vi "Registry Set.vi"() -> (0 "error out":errorcluster)   [LabVIEW 2012]
uses:
  <vilib>/Rock Robotics/WPI/Joystick/WPI_JoystickDeviceEnum.ctl
  <vilib>/Rock Robotics/SystemInterfaces/AI/FPGA_AIChannel.ctl
  <vilib>/Rock Robotics/SystemInterfaces/Typedef/FPGA_TypedefAnalogModule.ctl
  <vilib>/Rock Robotics/SystemInterfaces/DIO/FPGA_DIOPWMChannel.ctl
  <vilib>/Rock Robotics/SystemInterfaces/Typedef/FPGA_TypedefDigitalModule.ctl
  <vilib>/Rock Robotics/SystemInterfaces/DIO/FPGA_DIOChannel.ctl
  <vilib>/Rock Robotics/SystemInterfaces/DIO/FPGA_DIORelayChannel.ctl
  <vilib>/Rock Robotics/WPI/Solenoid/WPI_SolenoidChannel.ctl
  <vilib>/Rock Robotics/SystemInterfaces/Typedef/FPGA_TypedefSolenoidModule.ctl
  <vilib>/Rock Robotics/WPI/MotorControl/WPI_MotorControlOpen Talon.vi
  <vilib>/Rock Robotics/WPI/Solenoid/WPI_SolenoidOpenSingle.vi
  <vilib>/Rock Robotics/WPI/Solenoid/WPI_SolenoidOpenDouble.vi
  Global Refnums.vi
  <vilib>/Rock Robotics/WPI/Compressor/WPI_CompressorGetSetRefNum.vi
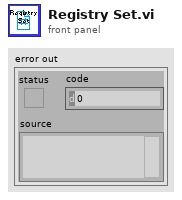
[diagram p1: front panel]
types:
  T1 = typedef "WPI_SolenoidChannel.ctl" = enum8{"Solenoid 1", "Solenoid 2", "Solenoid 3", "Solenoid 4", "Solenoid 5", "Solenoid 6", "Solenoid 7", "Solenoid 8", "Invalid"}
  T2 = typedef "FPGA_TypedefSolenoidModule.ctl" = enum16{"Solenoid Module 1", "Solenoid Module 2"}
  T3 = typedef "FPGA_DIOChannel.ctl" = enum8{"DIO 1", "DIO 2", "DIO 3", "DIO 4", "DIO 5", "DIO 6", "DIO 7", "DIO 8", "DIO 9", "DIO 10", "DIO 11", "DIO 12", "DIO 13", "DIO 14", "Invalid"}
  T4 = typedef "FPGA_TypedefDigitalModule.ctl" = enum16{"Digital Module 1", "Digital Module 2"}
  T5 = typedef "FPGA_DIOPWMChannel.ctl" = enum8{"PWM 1", "PWM 2", "PWM 3", "PWM 4", "PWM 5", "PWM 6", "PWM 7", "PWM 8", "PWM 9", "PWM 10", "Invalid"}
  T6 = typedef "FPGA_DIORelayChannel.ctl" = enum8{"Relay 1", "Relay 2", "Relay 3", "Relay 4", "Relay 5", "Relay 6", "Relay 7", "Relay 8", "Invalid"}
  T7 = typedef "FPGA_AIChannel.ctl" = enum8{"AI 1", "AI 2", "AI 3", "AI 4", "AI 5", "AI 6", "AI 7", "AI 8", "Invalid"}
  T8 = typedef "FPGA_TypedefAnalogModule.ctl" = enum16{"Analog Module 1", "Analog Module 2"}
  T9 = typedef "WPI_JoystickDeviceEnum.ctl" = enum16{"USB 1", "USB 2", "USB 3", "USB 4", "Kinect 1", "Kinect 2"}
  T10 = typedef "WPI_AnalogChannelDevRef.ctl" = cluster{"DevStatus":errorcluster, "Analog Module":T8, "Analog Channel":T7}
  T11 = typedef "WPI_JoystickDevRef.ctl" = cluster{"Device":T9}
  T12 = typedef "WPI_CompressorDevRef.ctl" = cluster{"DevStatus":errorcluster, "DigitalInputDevRef":T13, "RelayDevRef":T14}
  T13 = typedef "WPI_DigitalInputDevRef.ctl" = cluster{"DevStatus":errorcluster, "DIO Channel":T3, "Digital Module":T4}
  T14 = typedef "WPI_RelayDevRef.ctl" = cluster{"DevStatus":errorcluster, "Relay Channel":T6, "Digital Module":T4, "Relay Direction":T15}
  T15 = typedef "WPI_RelayDirection.ctl" = enum16{"Both directions", "Forward only", "Reverse only"}
  T16 = typedef "WPI_MotorControlDeviceRef.ctl" = cluster{"DeviceStatus":errorcluster, "Type":enum16{"PWM", "CAN"}, "PWM":cluster{"Digital Module":T4, "PWM Channel":T5, "DeadBand":T17}, "CAN":cluster{"Device Number":u8, "Control Mode":T18, "Semaphore":T19, "Max Vout":dbl}, "Invert":bool, "TransformRef":T20, "InvTransformRef":T20}
  T17 = typedef "WPI_PWMDeadband.ctl" = cluster{"Name":string, "maxPositivePwm":i32, "minPositivePwm":i32, "centerPwm":i32, "maxNegativePwm":i32, "minNegativePwm":i32, "angularRange":u16}
  T18 = typedef "WPI_CANJaguar_ControlMode.ctl" = enum8{"Percent VBus", "Current", "Speed", "Position", "Voltage"}
  T19 = typedef "Semaphore RefNum" = refnum<k1>
  T20 = typedef "WPI_PWMTransform_ConPane.ctl" = refnum<vi>
  T21 = typedef "WPI_SolenoidDevRef.ctl" = cluster{"DevStatus":errorcluster, "Solenoid Module":T2, "Forward Solenoid Channel":T1, "Reverse Solenoid Channel":T1}
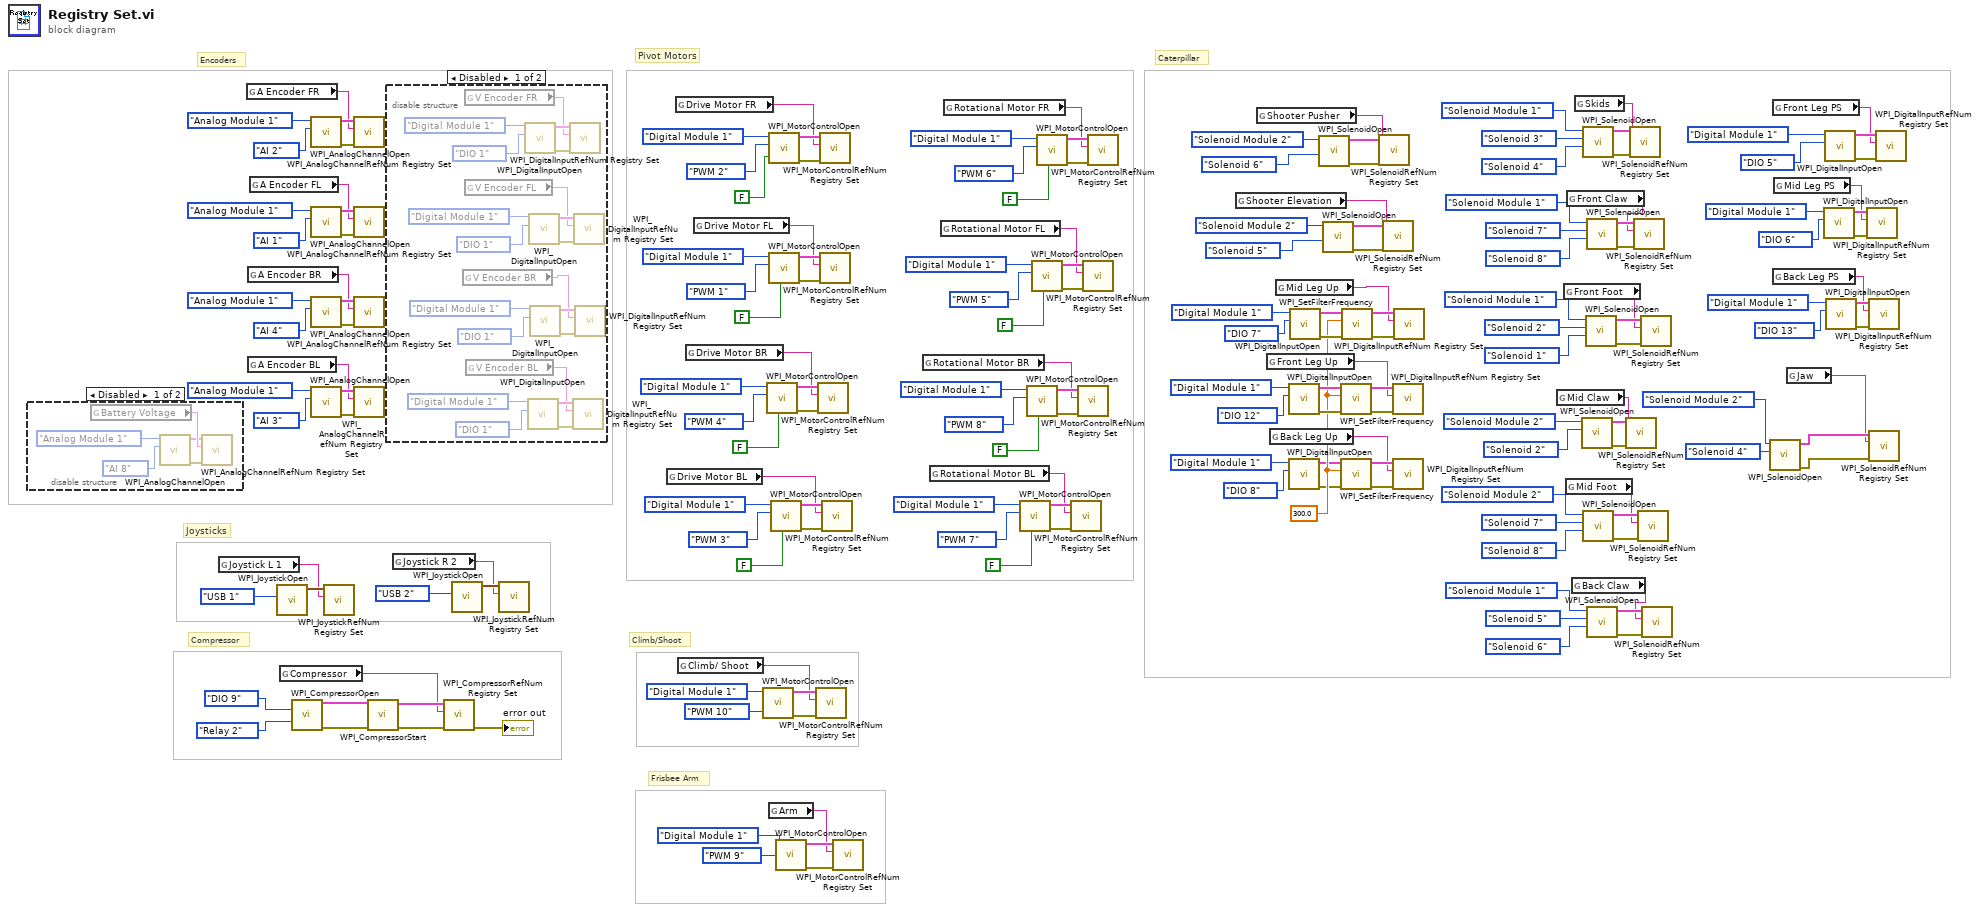
[diagram p0: block diagram]
diagram:
  w91 = 300.0 ("Filter Frequency")
  # "Frisbee Arm"
  # "Compressor"
  # "Climb/Shoot"
  # "Caterpillar"
  # "Pivot Motors"
  # "Encoders"
  # "Joysticks"
  n1 = disable-structure shown="Disabled" {
    frame Disabled {
      n2 = global read "Global Refnums.vi" "Battery Voltage"() -> (w184:string)
      n3 = call <vilib>:"WPI_AnalogChannelOpen.vi"("Analog Channel"=FPGA_AIChannel."AI 8", "Analog Module (Module 1)"=FPGA_TypedefAnalogModule."Analog Module 1") -> ("error out"=w181:errorcluster, "AIDeviceRef"=w180:T10)  [unwired: 8 in]
      n4 = call <vilib>:"WPI_AnalogChannelRefNum Registry Set.vi"("error in (no error)"=w181, "refnum name"=w184, "AIDeviceRef"=w180) -> ()  [unwired: 7 in, 2 out]
    }
    frame Enabled {
    }
  }
  n5 = global read "Global Refnums.vi" "Joystick L 1"() -> (w177:string)
  n6 = global read "Global Refnums.vi" "A Encoder FR"() -> (w169:string)
  n7 = global read "Global Refnums.vi" "A Encoder BR"() -> (w155:string)
  n8 = global read "Global Refnums.vi" "A Encoder BL"() -> (w154:string)
  n9 = global read "Global Refnums.vi" "A Encoder FL"() -> (w156:string)
  n10 = call <vilib>:"WPI_JoystickOpen.vi"("JoystickDevice"=WPI_JoystickDeviceEnum."USB 1") -> ("JoystickDevRef"=w178:T11)  [unwired: 10 in]
  n11 = global read "Global Refnums.vi" "Compressor"() -> (w80:string)
  n12 = call <vilib>:"WPI_CompressorOpen.vi"("Pressure Switch DIO Channel"=FPGA_DIOChannel."DIO 9", "Relay Channel"=FPGA_DIORelayChannel."Relay 2") -> ("CompressorDevRef"=w86:T12, "error out"=w85:errorcluster)  [unwired: 12 in]
  n13 = call <vilib>:"WPI_AnalogChannelOpen.vi"("Analog Channel"=FPGA_AIChannel."AI 2", "Analog Module (Module 1)"=FPGA_TypedefAnalogModule."Analog Module 1") -> ("error out"=w172:errorcluster, "AIDeviceRef"=w173:T10)  [unwired: 8 in]
  n14 = call <vilib>:"WPI_AnalogChannelOpen.vi"("Analog Channel"=FPGA_AIChannel."AI 1", "Analog Module (Module 1)"=FPGA_TypedefAnalogModule."Analog Module 1") -> ("error out"=w167:errorcluster, "AIDeviceRef"=w168:T10)  [unwired: 8 in]
  n15 = call <vilib>:"WPI_AnalogChannelOpen.vi"("Analog Channel"=FPGA_AIChannel."AI 4", "Analog Module (Module 1)"=FPGA_TypedefAnalogModule."Analog Module 1") -> ("error out"=w163:errorcluster, "AIDeviceRef"=w164:T10)  [unwired: 8 in]
  n16 = call <vilib>:"WPI_AnalogChannelOpen.vi"("Analog Channel"=FPGA_AIChannel."AI 3", "Analog Module (Module 1)"=FPGA_TypedefAnalogModule."Analog Module 1") -> ("error out"=w159:errorcluster, "AIDeviceRef"=w160:T10)  [unwired: 8 in]
  n17 = call <vilib>:"WPI_JoystickRefNum Registry Set.vi"("refnum name"=w177, "JoystickDevRef"=w178) -> ()  [unwired: 8 in, 2 out]
  n18 = call <vilib>:"WPI_AnalogChannelRefNum Registry Set.vi"("error in (no error)"=w172, "refnum name"=w169, "AIDeviceRef"=w173) -> ()  [unwired: 7 in, 2 out]
  n19 = call <vilib>:"WPI_AnalogChannelRefNum Registry Set.vi"("error in (no error)"=w167, "refnum name"=w156, "AIDeviceRef"=w168) -> ()  [unwired: 7 in, 2 out]
  n20 = call <vilib>:"WPI_AnalogChannelRefNum Registry Set.vi"("error in (no error)"=w163, "refnum name"=w155, "AIDeviceRef"=w164) -> ()  [unwired: 7 in, 2 out]
  n21 = call <vilib>:"WPI_AnalogChannelRefNum Registry Set.vi"("error in (no error)"=w159, "refnum name"=w154, "AIDeviceRef"=w160) -> ()  [unwired: 7 in, 2 out]
  n22 = call <vilib>:"WPI_CompressorStart.vi"("error in (no error)"=w85, "CompressorDevRef"=w86) -> ("error out"=w83:errorcluster, "CompressorDevRef"=w84:T12)  [unwired: 8 in]
  n23 = disable-structure shown="Disabled" {
    frame Disabled {
      n24 = global read "Global Refnums.vi" "V Encoder BR"() -> (w190:string)
      n25 = global read "Global Refnums.vi" "V Encoder FR"() -> (w202:string)
      n26 = global read "Global Refnums.vi" "V Encoder FL"() -> (w195:string)
      n27 = global read "Global Refnums.vi" "V Encoder BL"() -> (w185:string)
      n28 = call <vilib>:"WPI_DigitalInputOpen.vi"("DIO Channel"=FPGA_DIOChannel."DIO 1", "Digital Module (Module 1)"=FPGA_TypedefDigitalModule."Digital Module 1") -> ("error out"=w204:errorcluster, "DigitalInputDevRef"=w203:T13)  [unwired: 8 in]
      n29 = call <vilib>:"WPI_DigitalInputOpen.vi"("DIO Channel"=FPGA_DIOChannel."DIO 1", "Digital Module (Module 1)"=FPGA_TypedefDigitalModule."Digital Module 1") -> ("error out"=w189:errorcluster, "DigitalInputDevRef"=w188:T13)  [unwired: 8 in]
      n30 = call <vilib>:"WPI_DigitalInputOpen.vi"("DIO Channel"=FPGA_DIOChannel."DIO 1", "Digital Module (Module 1)"=FPGA_TypedefDigitalModule."Digital Module 1") -> ("error out"=w199:errorcluster, "DigitalInputDevRef"=w198:T13)  [unwired: 8 in]
      n31 = call <vilib>:"WPI_DigitalInputOpen.vi"("DIO Channel"=FPGA_DIOChannel."DIO 1", "Digital Module (Module 1)"=FPGA_TypedefDigitalModule."Digital Module 1") -> ("error out"=w194:errorcluster, "DigitalInputDevRef"=w193:T13)  [unwired: 8 in]
      n32 = call <vilib>:"WPI_DigitalInputRefNum Registry Set.vi"("error in (no error)"=w204, "refnum name"=w202, "DigitalInputDevRef"=w203) -> ()  [unwired: 7 in, 2 out]
      n33 = call <vilib>:"WPI_DigitalInputRefNum Registry Set.vi"("error in (no error)"=w189, "refnum name"=w185, "DigitalInputDevRef"=w188) -> ()  [unwired: 7 in, 2 out]
      n34 = call <vilib>:"WPI_DigitalInputRefNum Registry Set.vi"("error in (no error)"=w199, "refnum name"=w195, "DigitalInputDevRef"=w198) -> ()  [unwired: 7 in, 2 out]
      n35 = call <vilib>:"WPI_DigitalInputRefNum Registry Set.vi"("error in (no error)"=w194, "refnum name"=w190, "DigitalInputDevRef"=w193) -> ()  [unwired: 7 in, 2 out]
    }
    frame Enabled {
    }
  }
  n36 = global read "Global Refnums.vi" "Joystick R 2"() -> (w174:string)
  n37 = call <vilib>:"WPI_CompressorRefNum Registry Set.vi"("error in (no error)"=w83, "refnum name"=w80, "CompressorDevRef"=w84) -> ("error out"=→"error out":errorcluster)  [unwired: 7 in, 1 out]
  n38 = call <vilib>:"WPI_JoystickOpen.vi"("JoystickDevice"=WPI_JoystickDeviceEnum."USB 2") -> ("JoystickDevRef"=w175:T11)  [unwired: 10 in]
  n39 = call <vilib>:"WPI_JoystickRefNum Registry Set.vi"("refnum name"=w174, "JoystickDevRef"=w175) -> ()  [unwired: 8 in, 2 out]
  n40 = global read "Global Refnums.vi" "Drive Motor BL"() -> (w131:string)
  n41 = global read "Global Refnums.vi" "Drive Motor FR"() -> (w149:string)
  n42 = global read "Global Refnums.vi" "Climb/ Shoot"() -> (w32:string)
  n43 = global read "Global Refnums.vi" "Drive Motor BR"() -> (w130:string)
  n44 = global read "Global Refnums.vi" "Drive Motor FL"() -> (w137:string)
  n45 = call-poly <vilib>:"WPI_MotorControlOpen.vi"("PWM Channel"=FPGA_DIOPWMChannel."PWM 10", "Digital Module (Module 1)"=FPGA_TypedefDigitalModule."Digital Module 1") -> ("error out"=w35:errorcluster, "MotorControlDeviceRef"=w36:T16)  [unwired: 8 in]
  n46 = call-poly <vilib>:"WPI_MotorControlOpen.vi"("Invert"=FALSE, "PWM Channel"=FPGA_DIOPWMChannel."PWM 4", "Digital Module (Module 1)"=FPGA_TypedefDigitalModule."Digital Module 1") -> ("error out"=w139:errorcluster, "MotorControlDeviceRef"=w140:T16)  [unwired: 7 in]
  n47 = call-poly <vilib>:"WPI_MotorControlOpen.vi"("Invert"=FALSE, "PWM Channel"=FPGA_DIOPWMChannel."PWM 2", "Digital Module (Module 1)"=FPGA_TypedefDigitalModule."Digital Module 1") -> ("error out"=w150:errorcluster, "MotorControlDeviceRef"=w151:T16)  [unwired: 7 in]
  n48 = call-poly <vilib>:"WPI_MotorControlOpen.vi"("Invert"=FALSE, "PWM Channel"=FPGA_DIOPWMChannel."PWM 1", "Digital Module (Module 1)"=FPGA_TypedefDigitalModule."Digital Module 1") -> ("error out"=w144:errorcluster, "MotorControlDeviceRef"=w145:T16)  [unwired: 7 in]
  n49 = global read "Global Refnums.vi" "Arm"() -> (w18:string)
  n50 = call-poly <vilib>:"WPI_MotorControlOpen.vi"("Invert"=FALSE, "PWM Channel"=FPGA_DIOPWMChannel."PWM 3", "Digital Module (Module 1)"=FPGA_TypedefDigitalModule."Digital Module 1") -> ("error out"=w133:errorcluster, "MotorControlDeviceRef"=w134:T16)  [unwired: 7 in]
  n51 = call-poly <vilib>:"WPI_MotorControlOpen.vi"("PWM Channel"=FPGA_DIOPWMChannel."PWM 9", "Digital Module (Module 1)"=FPGA_TypedefDigitalModule."Digital Module 1") -> ("error out"=w20:errorcluster, "MotorControlDeviceRef"=w19:T16)  [unwired: 8 in]
  n52 = call <vilib>:"WPI_MotorControlRefNum Registry Set.vi"("error in (no error)"=w35, "refnum name"=w32, "MotorControlDevRef"=w36) -> ()  [unwired: 7 in, 2 out]
  n53 = call <vilib>:"WPI_MotorControlRefNum Registry Set.vi"("error in (no error)"=w139, "refnum name"=w130, "MotorControlDevRef"=w140) -> ()  [unwired: 7 in, 2 out]
  n54 = call <vilib>:"WPI_MotorControlRefNum Registry Set.vi"("error in (no error)"=w150, "refnum name"=w149, "MotorControlDevRef"=w151) -> ()  [unwired: 7 in, 2 out]
  n55 = call <vilib>:"WPI_MotorControlRefNum Registry Set.vi"("error in (no error)"=w144, "refnum name"=w137, "MotorControlDevRef"=w145) -> ()  [unwired: 7 in, 2 out]
  n56 = call <vilib>:"WPI_MotorControlRefNum Registry Set.vi"("error in (no error)"=w133, "refnum name"=w131, "MotorControlDevRef"=w134) -> ()  [unwired: 7 in, 2 out]
  n57 = call <vilib>:"WPI_MotorControlRefNum Registry Set.vi"("error in (no error)"=w20, "refnum name"=w18, "MotorControlDevRef"=w19) -> ()  [unwired: 7 in, 2 out]
  n58 = global read "Global Refnums.vi" "Rotational Motor BR"() -> (w109:string)
  n59 = global read "Global Refnums.vi" "Rotational Motor BL"() -> (w106:string)
  n60 = global read "Global Refnums.vi" "Rotational Motor FL"() -> (w108:string)
  n61 = global read "Global Refnums.vi" "Rotational Motor FR"() -> (w107:string)
  n62 = call-poly <vilib>:"WPI_MotorControlOpen.vi"("Invert"=FALSE, "PWM Channel"=FPGA_DIOPWMChannel."PWM 7", "Digital Module (Module 1)"=FPGA_TypedefDigitalModule."Digital Module 1") -> ("error out"=w111:errorcluster, "MotorControlDeviceRef"=w112:T16)  [unwired: 7 in]
  n63 = call-poly <vilib>:"WPI_MotorControlOpen.vi"("Invert"=FALSE, "PWM Channel"=FPGA_DIOPWMChannel."PWM 8", "Digital Module (Module 1)"=FPGA_TypedefDigitalModule."Digital Module 1") -> ("error out"=w116:errorcluster, "MotorControlDeviceRef"=w117:T16)  [unwired: 7 in]
  n64 = call-poly <vilib>:"WPI_MotorControlOpen.vi"("Invert"=FALSE, "PWM Channel"=FPGA_DIOPWMChannel."PWM 5", "Digital Module (Module 1)"=FPGA_TypedefDigitalModule."Digital Module 1") -> ("error out"=w121:errorcluster, "MotorControlDeviceRef"=w122:T16)  [unwired: 7 in]
  n65 = call-poly <vilib>:"WPI_MotorControlOpen.vi"("Invert"=FALSE, "PWM Channel"=FPGA_DIOPWMChannel."PWM 6", "Digital Module (Module 1)"=FPGA_TypedefDigitalModule."Digital Module 1") -> ("error out"=w126:errorcluster, "MotorControlDeviceRef"=w127:T16)  [unwired: 7 in]
  n66 = call <vilib>:"WPI_MotorControlRefNum Registry Set.vi"("error in (no error)"=w111, "refnum name"=w106, "MotorControlDevRef"=w112) -> ()  [unwired: 7 in, 2 out]
  n67 = call <vilib>:"WPI_MotorControlRefNum Registry Set.vi"("error in (no error)"=w116, "refnum name"=w109, "MotorControlDevRef"=w117) -> ()  [unwired: 7 in, 2 out]
  n68 = call <vilib>:"WPI_MotorControlRefNum Registry Set.vi"("error in (no error)"=w121, "refnum name"=w108, "MotorControlDevRef"=w122) -> ()  [unwired: 7 in, 2 out]
  n69 = call <vilib>:"WPI_MotorControlRefNum Registry Set.vi"("error in (no error)"=w126, "refnum name"=w107, "MotorControlDevRef"=w127) -> ()  [unwired: 7 in, 2 out]
  n70 = global read "Global Refnums.vi" "Shooter Elevation"() -> (w70:string)
  n71 = global read "Global Refnums.vi" "Shooter Pusher"() -> (w69:string)
  n72 = global read "Global Refnums.vi" "Front Leg Up"() -> (w30:string)
  n73 = global read "Global Refnums.vi" "Back Leg Up"() -> (w29:string)
  n74 = global read "Global Refnums.vi" "Mid Leg Up"() -> (w31:string)
  n75 = call <vilib>:"WPI_DigitalInputOpen.vi"("DIO Channel"=FPGA_DIOChannel."DIO 12", "Digital Module (Module 1)"=FPGA_TypedefDigitalModule."Digital Module 1") -> ("error out"=w93:errorcluster, "DigitalInputDevRef"=w94:T13)  [unwired: 8 in]
  n76 = call <vilib>:"WPI_DigitalInputOpen.vi"("DIO Channel"=FPGA_DIOChannel."DIO 8", "Digital Module (Module 1)"=FPGA_TypedefDigitalModule."Digital Module 1") -> ("error out"=w90:errorcluster, "DigitalInputDevRef"=w89:T13)  [unwired: 8 in]
  n77 = call <vilib>:"WPI_DigitalInputOpen.vi"("DIO Channel"=FPGA_DIOChannel."DIO 7", "Digital Module (Module 1)"=FPGA_TypedefDigitalModule."Digital Module 1") -> ("error out"=w98:errorcluster, "DigitalInputDevRef"=w99:T13)  [unwired: 8 in]
  n78 = call-poly <vilib>:"WPI_SolenoidOpen.vi"("Solenoid Channel"=WPI_SolenoidChannel."Solenoid 6", "Solenoid Module (Module 1)"=FPGA_TypedefSolenoidModule."Solenoid Module 2") -> ("error out"=w75:errorcluster, "SolenoidDevRef"=w76:T21)  [unwired: 8 in]
  n79 = call-poly <vilib>:"WPI_SolenoidOpen.vi"("Solenoid Channel"=WPI_SolenoidChannel."Solenoid 5", "Solenoid Module (Module 1)"=FPGA_TypedefSolenoidModule."Solenoid Module 2") -> ("error out"=w71:errorcluster, "SolenoidDevRef"=w72:T21)  [unwired: 8 in]
  n80 = call <vilib>:"WPI_SetFilterFrequency.vi"("error in (no error)"=w93, "Filter Frequency"=w91, "DigitalInputDevRef"=w94) -> ("error out"=w92:errorcluster, "DigitalInputDevRef"=w95:T13)  [unwired: 7 in]
  n81 = call <vilib>:"WPI_SetFilterFrequency.vi"("error in (no error)"=w90, "Filter Frequency"=w91, "DigitalInputDevRef"=w89) -> ("error out"=w87:errorcluster, "DigitalInputDevRef"=w88:T13)  [unwired: 7 in]
  n82 = call <vilib>:"WPI_SetFilterFrequency.vi"("error in (no error)"=w98, "Filter Frequency"=w91, "DigitalInputDevRef"=w99) -> ("error out"=w96:errorcluster, "DigitalInputDevRef"=w97:T13)  [unwired: 7 in]
  n83 = call <vilib>:"WPI_SolenoidRefNum Registry Set.vi"("error in (no error)"=w75, "refnum name"=w69, "SolenoidDevRef"=w76) -> ()  [unwired: 7 in, 2 out]
  n84 = call <vilib>:"WPI_SolenoidRefNum Registry Set.vi"("error in (no error)"=w71, "refnum name"=w70, "SolenoidDevRef"=w72) -> ()  [unwired: 7 in, 2 out]
  n85 = call <vilib>:"WPI_DigitalInputRefNum Registry Set.vi"("error in (no error)"=w92, "refnum name"=w30, "DigitalInputDevRef"=w95) -> ()  [unwired: 7 in, 2 out]
  n86 = call <vilib>:"WPI_DigitalInputRefNum Registry Set.vi"("error in (no error)"=w87, "refnum name"=w29, "DigitalInputDevRef"=w88) -> ()  [unwired: 7 in, 2 out]
  n87 = call <vilib>:"WPI_DigitalInputRefNum Registry Set.vi"("error in (no error)"=w96, "refnum name"=w31, "DigitalInputDevRef"=w97) -> ()  [unwired: 7 in, 2 out]
  n88 = global read "Global Refnums.vi" "Mid Claw"() -> (w2:string)
  n89 = global read "Global Refnums.vi" "Front Foot"() -> (w26:string)
  n90 = global read "Global Refnums.vi" "Mid Foot"() -> (w7:string)
  n91 = global read "Global Refnums.vi" "Front Claw"() -> (w28:string)
  n92 = global read "Global Refnums.vi" "Back Claw"() -> (w25:string)
  n93 = global read "Global Refnums.vi" "Skids"() -> (w27:string)
  n94 = call-poly <vilib>:"WPI_SolenoidOpen.vi"("Solenoid Channel"=WPI_SolenoidChannel."Solenoid 2", "Solenoid Module (Module 1)"=FPGA_TypedefSolenoidModule."Solenoid Module 2") -> ("error out"=w61:errorcluster, "SolenoidDevRef"=w62:T21)  [unwired: 8 in]
  n95 = call-poly <vilib>:"WPI_SolenoidOpen.vi"("Reverse Solenoid Channel"=WPI_SolenoidChannel."Solenoid 4", "Forward Solenoid Channel"=WPI_SolenoidChannel."Solenoid 3" ("Solenoid Channel"), "Solenoid Module (Module 1)"=FPGA_TypedefSolenoidModule."Solenoid Module 1") -> ("error out"=w48:errorcluster, "SolenoidDevRef"=w49:T21)  [unwired: 7 in]
  n96 = call-poly <vilib>:"WPI_SolenoidOpen.vi"("Reverse Solenoid Channel"=WPI_SolenoidChannel."Solenoid 8", "Forward Solenoid Channel"=WPI_SolenoidChannel."Solenoid 7", "Solenoid Module (Module 1)"=FPGA_TypedefSolenoidModule."Solenoid Module 2") -> ("error out"=w8:errorcluster, "SolenoidDevRef"=w12:T21)  [unwired: 7 in]
  n97 = call-poly <vilib>:"WPI_SolenoidOpen.vi"("Reverse Solenoid Channel"=WPI_SolenoidChannel."Solenoid 1", "Forward Solenoid Channel"=WPI_SolenoidChannel."Solenoid 2", "Solenoid Module (Module 1)"=FPGA_TypedefSolenoidModule."Solenoid Module 1") -> ("error out"=w52:errorcluster, "SolenoidDevRef"=w56:T21)  [unwired: 7 in]
  n98 = call-poly <vilib>:"WPI_SolenoidOpen.vi"("Reverse Solenoid Channel"=WPI_SolenoidChannel."Solenoid 8", "Forward Solenoid Channel"=WPI_SolenoidChannel."Solenoid 7" ("Solenoid Channel"), "Solenoid Module (Module 1)"=FPGA_TypedefSolenoidModule."Solenoid Module 1") -> ("error out"=w65:errorcluster, "SolenoidDevRef"=w66:T21)  [unwired: 7 in]
  n99 = call-poly <vilib>:"WPI_SolenoidOpen.vi"("Reverse Solenoid Channel"=WPI_SolenoidChannel."Solenoid 6", "Forward Solenoid Channel"=WPI_SolenoidChannel."Solenoid 5" ("Solenoid Channel"), "Solenoid Module (Module 1)"=FPGA_TypedefSolenoidModule."Solenoid Module 1") -> ("error out"=w57:errorcluster, "SolenoidDevRef"=w58:T21)  [unwired: 7 in]
  n100 = call <vilib>:"WPI_SolenoidRefNum Registry Set.vi"("error in (no error)"=w61, "refnum name"=w2, "SolenoidDevRef"=w62) -> ()  [unwired: 7 in, 2 out]
  n101 = call <vilib>:"WPI_SolenoidRefNum Registry Set.vi"("error in (no error)"=w48, "refnum name"=w27, "SolenoidDevRef"=w49) -> ()  [unwired: 7 in, 2 out]
  n102 = call <vilib>:"WPI_SolenoidRefNum Registry Set.vi"("error in (no error)"=w65, "refnum name"=w28, "SolenoidDevRef"=w66) -> ()  [unwired: 7 in, 2 out]
  n103 = call <vilib>:"WPI_SolenoidRefNum Registry Set.vi"("error in (no error)"=w8, "refnum name"=w7, "SolenoidDevRef"=w12) -> ()  [unwired: 7 in, 2 out]
  n104 = call <vilib>:"WPI_SolenoidRefNum Registry Set.vi"("error in (no error)"=w52, "refnum name"=w26, "SolenoidDevRef"=w56) -> ()  [unwired: 7 in, 2 out]
  n105 = call <vilib>:"WPI_SolenoidRefNum Registry Set.vi"("error in (no error)"=w57, "refnum name"=w25, "SolenoidDevRef"=w58) -> ()  [unwired: 7 in, 2 out]
  n106 = call-poly <vilib>:"WPI_SolenoidOpen.vi"("Solenoid Channel"=WPI_SolenoidChannel."Solenoid 4", "Solenoid Module (Module 1)"=FPGA_TypedefSolenoidModule."Solenoid Module 2") -> ("error out"=w5:errorcluster, "SolenoidDevRef"=w6:T21)  [unwired: 8 in]
  n107 = global read "Global Refnums.vi" "Front Leg PS"() -> (w24:string)
  n108 = global read "Global Refnums.vi" "Back Leg PS"() -> (w13:string)
  n109 = global read "Global Refnums.vi" "Mid Leg PS"() -> (w23:string)
  n110 = global read "Global Refnums.vi" "Jaw"() -> (w1:string)
  n111 = call <vilib>:"WPI_DigitalInputOpen.vi"("DIO Channel"=FPGA_DIOChannel."DIO 6", "Digital Module (Module 1)"=FPGA_TypedefDigitalModule."Digital Module 1") -> ("error out"=w38:errorcluster, "DigitalInputDevRef"=w41:T13)  [unwired: 8 in]
  n112 = call <vilib>:"WPI_DigitalInputOpen.vi"("DIO Channel"=FPGA_DIOChannel."DIO 5", "Digital Module (Module 1)"=FPGA_TypedefDigitalModule."Digital Module 1") -> ("error out"=w37:errorcluster, "DigitalInputDevRef"=w42:T13)  [unwired: 8 in]
  n113 = call <vilib>:"WPI_DigitalInputOpen.vi"("DIO Channel"=FPGA_DIOChannel."DIO 13", "Digital Module (Module 1)"=FPGA_TypedefDigitalModule."Digital Module 1") -> ("error out"=w14:errorcluster, "DigitalInputDevRef"=w17:T13)  [unwired: 8 in]
  n114 = call <vilib>:"WPI_DigitalInputRefNum Registry Set.vi"("error in (no error)"=w38, "refnum name"=w23, "DigitalInputDevRef"=w41) -> ()  [unwired: 7 in, 2 out]
  n115 = call <vilib>:"WPI_DigitalInputRefNum Registry Set.vi"("error in (no error)"=w14, "refnum name"=w13, "DigitalInputDevRef"=w17) -> ()  [unwired: 7 in, 2 out]
  n116 = call <vilib>:"WPI_SolenoidRefNum Registry Set.vi"("error in (no error)"=w5, "refnum name"=w1, "SolenoidDevRef"=w6) -> ()  [unwired: 7 in, 2 out]
  n117 = call <vilib>:"WPI_DigitalInputRefNum Registry Set.vi"("error in (no error)"=w37, "refnum name"=w24, "DigitalInputDevRef"=w42) -> ()  [unwired: 7 in, 2 out]
